vi "Execute Initial Value Policy.vi"(8 "error in (no error)":errorcluster, 9 "Last Publish Time":timestamp, 10 "Last Topic Value":variant, 11 "ISubscriptionPolicy In":refnum<class "ISubscriptionPolicy.lvclass">) -> (0 "error out":errorcluster, 3 "ISubscriptionPolicy Out":refnum<class "ISubscriptionPolicy.lvclass">)   [LabVIEW 2020, in "MVA Framework.lvlib" / "IMediator.lvlib" / "ISubscriptionPolicy.lvclass"]
doc: "执行初始值策略"
uses:
  ISubscriptionPolicy.lvclass
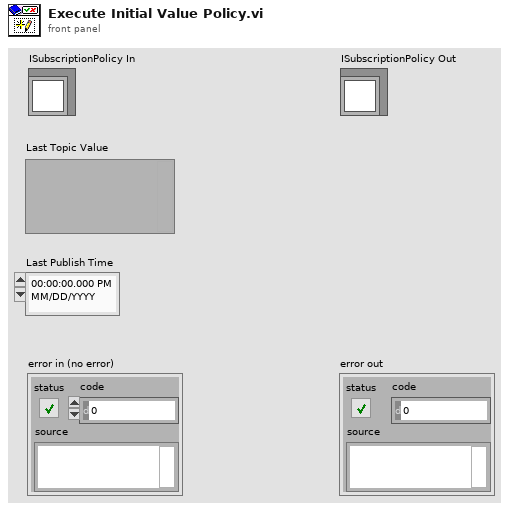
[diagram p1: front panel]
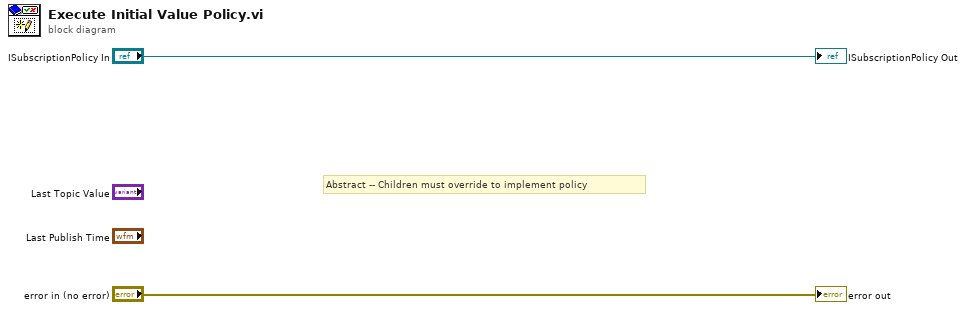
[diagram p0: block diagram]
diagram:
  # "Abstract -- Children must override to implement policy"
  "error out" <- "error in (no error)"
  "ISubscriptionPolicy Out" <- "ISubscriptionPolicy In"
